vi "Get Init Motor Data.vi"(8 "error in (no error)":errorcluster, 11 "SGDV_Ctrl_Class in":refnum<class "SGDV_Ctrl_Class.lvclass">) -> (0 "error out":errorcluster, 2 "Init Motor Data":T1, 3 "SGDV_Ctrl_Class out":refnum<class "SGDV_Ctrl_Class.lvclass">)   [LabVIEW 2013, in "SGDV_Ctrl_v13_lib.lvlib" / "SGDV_Ctrl_Class.lvclass"]
uses:
  SGDV_Ctrl_Class.lvclass
  Controls and General VIs/Init Motor Data.ctl
  SGDV_Ctrl_Class.lvclass/SGDV_Ctrl_Class.ctl
  SGDV_Ctrl_v13_lib.lvlib
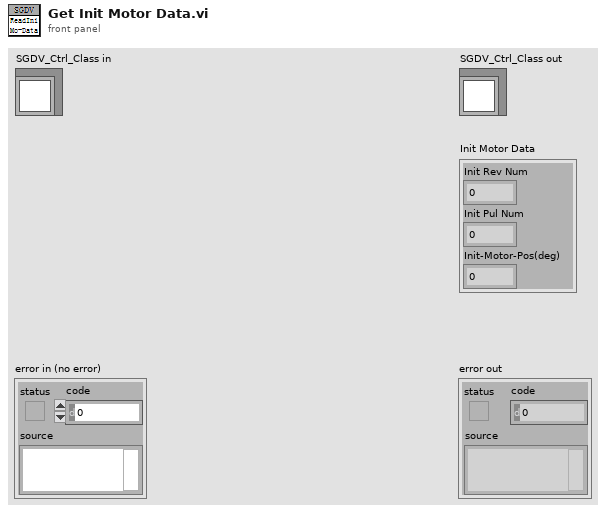
[diagram p1: front panel]
types:
  T1 = typedef "SGDV_Ctrl_v13_lib.lvlib/Init Motor Data.ctl" = cluster{"Init Rev Num":i32, "Init Pul Num":i32, "Init-Motor-Pos(deg)":dbl}
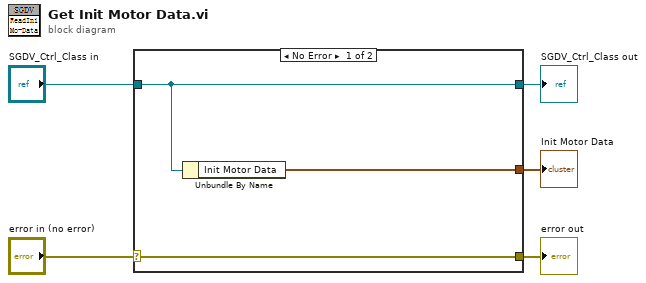
[diagram p0: block diagram]
diagram:
  n1 = case shown="No Error" "error in (no error)" {
    selector: "error in (no error)" -> [w8 w9]
    tunnel: [w8 w9] -> w4
    tunnel: [w7 w10] -> w2
    tunnel: "SGDV_Ctrl_Class in" -> [w7 w10]
    tunnel: [w6 _] -> w1
    frame No Error {
      n2 = Unbundle By Name(w7) -> ("Init Motor Data"=w6:T1)
    }
    frame Error {
    }
  }
  "error out" <- w4
  "SGDV_Ctrl_Class out" <- w2
  "Init Motor Data" <- w1
